vi "Test Error.vi"(11 "Test Case In":refnum<class "Error.lvclass">) -> (0 "error out":errorcluster, 3 "Test Case Out":refnum<class "Error.lvclass">)   [LabVIEW 2020, in "Error.lvclass"]
uses:
  Error.lvclass
  C:/git/astemes-lunit/source/LUnit Test Case.lvclass
  source/LUnit Test Case.lvclass/LUnit Test Case.ctl
  e14b8b0a-9b7b-4cf5-9f85-09c4314edb9a.vi
  source/Core/LUnit Test Case/Private/Append Pass Result.vi
  source/Core/LUnit Test Case/Private/Append Fail Result.vi
  e14b8b0a-9b7b-4cf5-9f85-09c4314edb9a.vi/9c5d11cd-9439-4240-a1ee-d9baace9c924.vi
  source/Core/LUnit Test Case/Private/Run In UI.vi
  <vilib>/Utility/error.llb/Clear Errors.vi
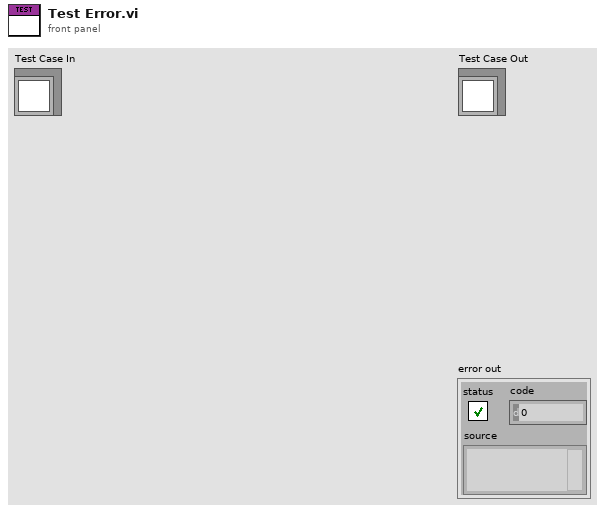
[diagram p1: front panel]
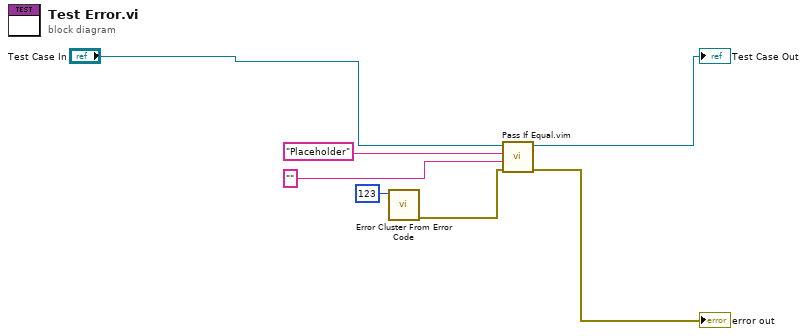
[diagram p0: block diagram]
diagram:
  n1 = call <vilib>:"Error Cluster From Error Code.vi"("error code (0)"=123) -> ("error out"=w2:errorcluster)  [unwired: 8 in]
  n2 = call "Pass If Equal.vim"("error in (no error)"=w2, "Actual"="", "Expected"="Placeholder", "LUnit Test Case In"="Test Case In") -> ("error out"=→"error out":errorcluster, "LUnit Test Case Out"=→"Test Case Out":refnum<class "Error.lvclass">)  [unwired: 6 in]
